vi "Close TCP.vi"(8 "error in":errorcluster) -> (0 "error out":errorcluster)   [LabVIEW 2017, in "WinHost.lvlib"]
uses:
  WinHost.lvlib
  Private TypeDefs/STM Queue Element.ctl
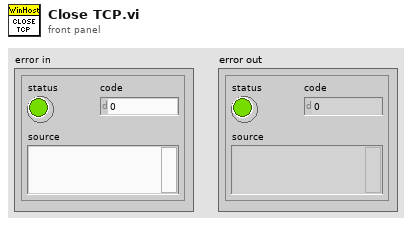
[diagram p1: front panel]
types:
  T1 = typedef "WinHost.lvlib/STM Queue Element.ctl" = cluster{"name":string, "data":string, "stop":bool}
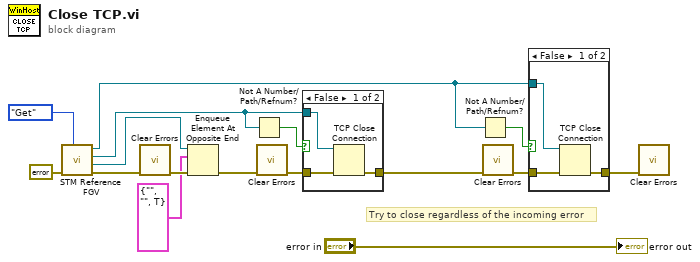
[diagram p0: block diagram]
diagram:
  # "Try to close regardless of the incoming error"
  n1 = call "STM Reference FGV.vi"("command"=enum16{"Set", "Get"}."Get", "error in"=errorcluster {"status"=FALSE, "code"=0, "source"=""}) -> ("error ou"=w4:errorcluster, "STM queue out"=w2:refnum<queue>, "TCP listener ID out"=w6:refnum<k5>, "TCP connection ID out"=w8:refnum<k5>)  [unwired: 6 in]
  n2 = call <vilib>:"Clear Errors.vi"("error in (no error)"=w4) -> ("error out"=w3:errorcluster)  [unwired: 5 in, 1 out]
  n3 = Enqueue Element At Opposite End(queue=w2, element=T1 {"name"="", "data"="", "stop"=TRUE}, error in (no error)=w3) -> (error out=w5:errorcluster)  [unwired: 1 in, 2 out]
  n4 = Not A Number/Path/Refnum?(number/path/refnum=w6) -> (NaN/Path/Refnum?=w14:bool)
  n5 = call <vilib>:"Clear Errors.vi"("error in (no error)"=w5) -> ("error out"=w15:errorcluster)  [unwired: 5 in, 1 out]
  n6 = case shown="False" w14 {
    tunnel: w15 -> [w19 w20]
    tunnel: w6 -> [w18 _]
    tunnel: [w17 w20] -> w9
    frame False {
      n7 = TCP Close Connection(connection ID=w18, error in (no error)=w19) -> (error out=w17:errorcluster)  [unwired: 1 in, 1 out]
    }
    frame True {
    }
  }
  n8 = Not A Number/Path/Refnum?(number/path/refnum=w8) -> (NaN/Path/Refnum?=w11:bool)
  n9 = call <vilib>:"Clear Errors.vi"("error in (no error)"=w9) -> ("error out"=w10:errorcluster)  [unwired: 5 in, 1 out]
  n10 = case shown="False" w11 {
    tunnel: w10 -> [w23 w24]
    tunnel: w8 -> [w22 _]
    tunnel: [w21 w24] -> w7
    frame False {
      n11 = TCP Close Connection(connection ID=w22, error in (no error)=w23) -> (error out=w21:errorcluster)  [unwired: 1 in, 1 out]
    }
    frame True {
    }
  }
  n12 = call <vilib>:"Clear Errors.vi"("error in (no error)"=w7) -> ()  [unwired: 5 in, 2 out]
  "error out" <- "error in"
